vi "Match Regular Expression.vi"() -> ()   [LabVIEW 2020]
uses:
  <vilib>/regexp/Match Regular Expression.xnode
panel:
  out "Expected Match":string[](array[string])
  out "Input String Length":i32
  out "Offset Past Match":i32[](array[numeric])
  out "Numeric":i32
  out "Extracted Number":dbl[](array[numeric])
  in  "String":string="Sita Ram Hanuman Sita Ram Hanuman Sita Ram Hanuman Sita Ram Hanuman Sita Ram Hanuman"
  # "OverView :"
  # "Note :"
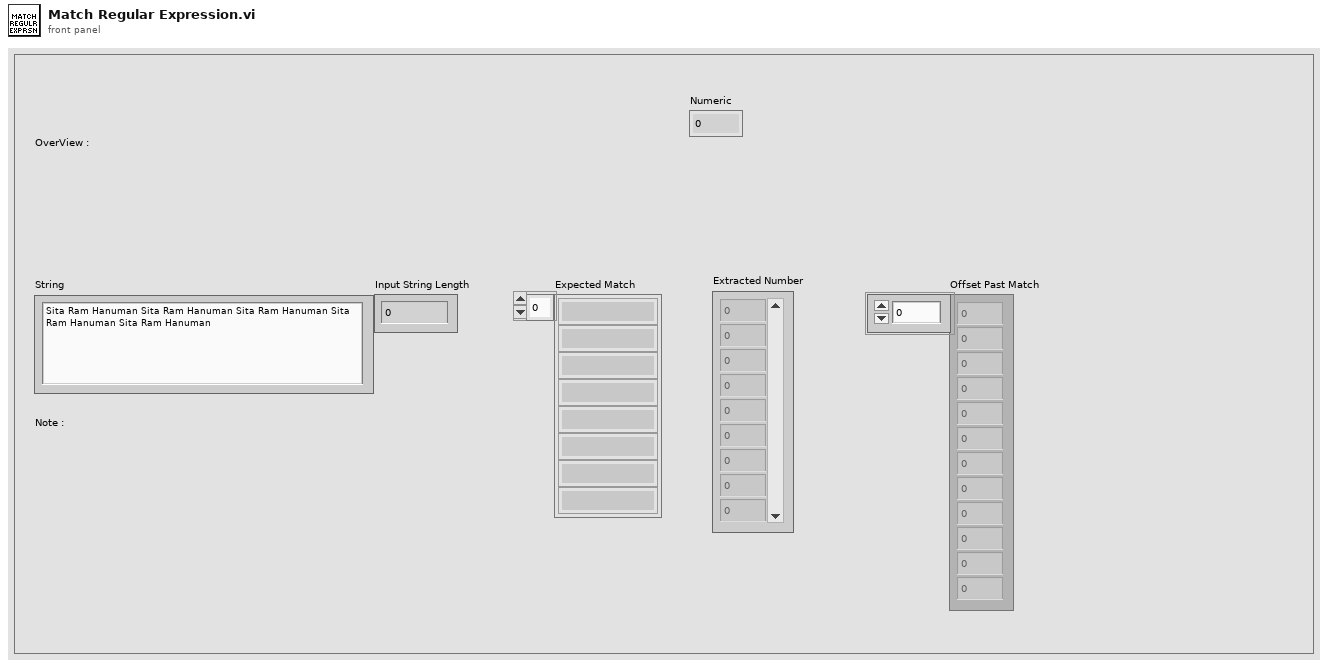
[diagram p1: front panel]
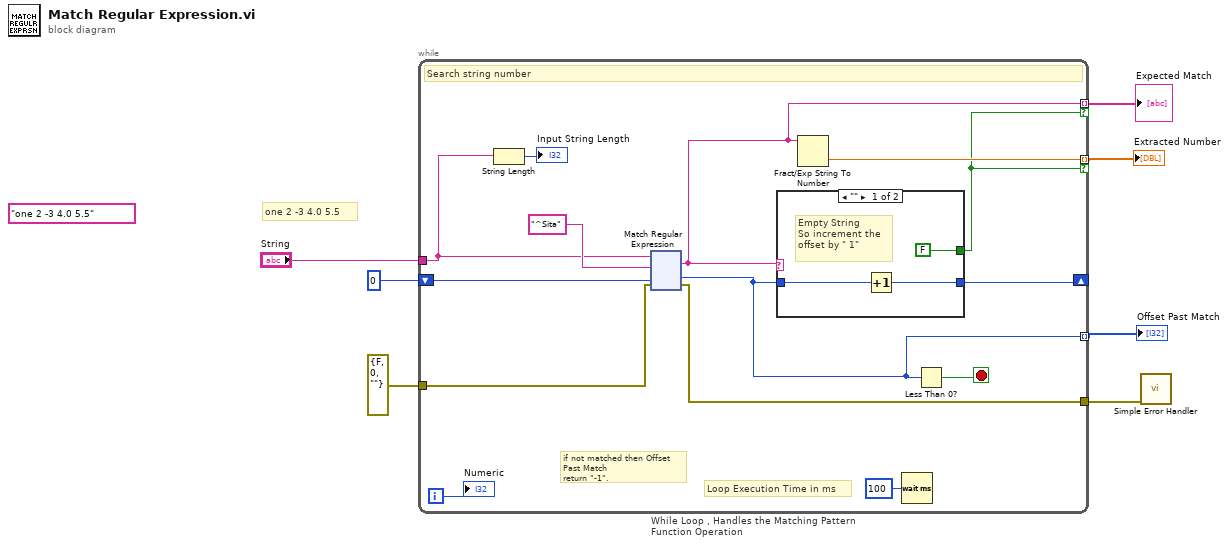
[diagram p0: block diagram]
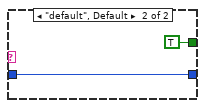
[diagram p2: hidden frame]
diagram:
  (unwired) "one 2 -3 4.0 5.5" ("String")
  # "one 2 -3 4.0 5.5"
  n1 = while "While Loop , Handles the Matching Pattern Function Operation" {
    tunnel: "String" -> [w12]
    shift-right: [w13] -> _
    shift-left: 0 -> [w20]
    tunnel: [w19] -> w5 mode=indexing if=w8
    tunnel: [w14] -> w4 mode=indexing
    tunnel: errorcluster {"status"=FALSE, "code"=0, "source"=""} ("error in") -> [w11]
    tunnel: [w10] -> w2
    tunnel: [w9] -> w1 mode=indexing if=w8
    i -> [w17]
    stop <- w15 stop-if-true
    # "Loop Execution Time in ms"
    # "if not matched then Offset Past Match\nreturn \"-1\"."
    # "Search string number"
    n2 = String Length(string=w12) -> (length=→"Input String Length":i32)
    n3 = xnode "Match Regular Expression"("input string"=w12, "regular expression"="^Sita", "offset (0)"=w20, "error in"=w11) -> ("whole match"=w9:string, "offset past match"=w14:i32, "error out"=w10:errorcluster)  [unwired: 2 in, 2 out]
    n4 = case shown="\"\"" w9 {
      tunnel: [w137 w139] -> w13
      tunnel: [FALSE TRUE] -> w8
      tunnel: w14 -> [w136 w139]
      frame "" {
        # "Empty String \nSo increment the \noffset by \" 1\""
        n5 = Increment(x=w136) -> (x+1=w137:i32)
      }
      frame "default", Default {
      }
    }
    n6 = Fract/Exp String To Number(string=w9) -> (number=w19:dbl)  [unwired: 3 in, 1 out]
    n7 = Wait (ms)(milliseconds to wait=u32 100) -> ()  [unwired: 1 out]
    n8 = Less Than 0?(x=w14) -> (x < 0?=w15:bool)
    "Numeric" <- w17
  }
  "Extracted Number" <- w5
  "Offset Past Match" <- w4
  "Expected Match" <- w1
  n9 = call <vilib>:"Simple Error Handler.vi"("error in (no error)"=w2) -> ()  [unwired: 4 in, 5 out]
